vi "UnloadCrvEdPanel.vi"(8 "error in (no error)":errorcluster caption="entrée d'erreur (pas d'erreur)", 10 "CrvEdViRef":refnum<vi>, 11 "RemPanRef":refnum<vi>) -> (0 "error out":errorcluster caption="sortie d'erreur")   [LabVIEW 2019]
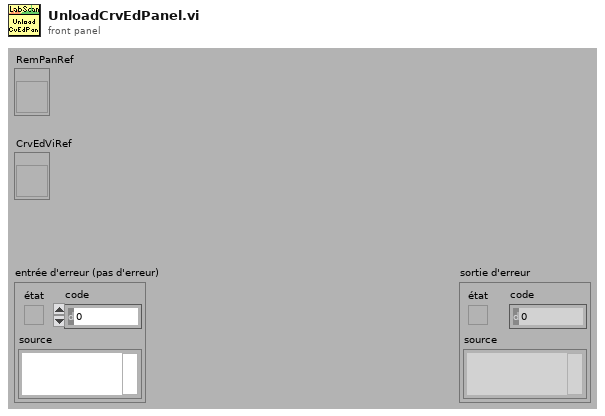
[diagram p1: front panel]
types:
  T1 = enum32{"Bad", "Idle", "Run top level", "Running"}
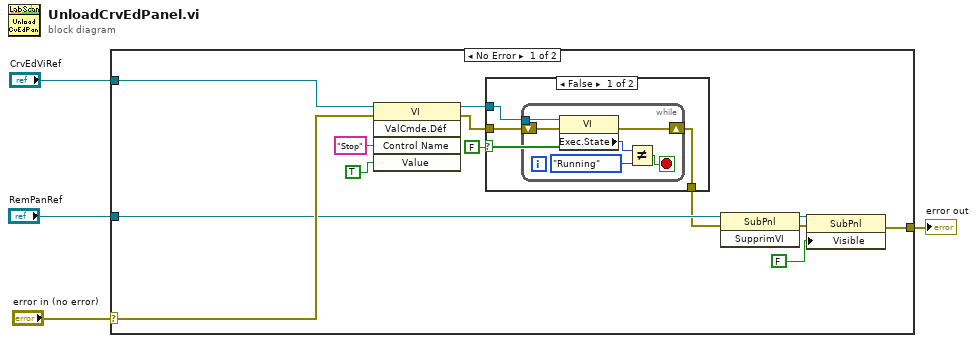
[diagram p0: block diagram]
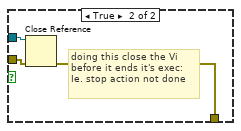
[diagram p2: hidden frame]
diagram:
  n1 = case shown="No Error" "error in (no error)" {
    selector: "error in (no error)" -> [w17 w30]
    tunnel: [w16 w30] -> w3
    tunnel: "RemPanRef" -> [w15 _]
    tunnel: "CrvEdViRef" -> [w14 _]
    frame No Error {
      n2 = invoke class="VI" method="ValCmde.Déf"(reference=w14, error in=w17, "Control Name"="Stop" ("Nom de la commande"), "Value"=TRUE) -> (reference out=w10:refnum<vi>, error out=w11:errorcluster)  [unwired: 1 in, 3 out]
      n3 = case shown="False" FALSE {
        tunnel: w11 -> [w19 w29]
        tunnel: w10 -> [w20 w28]
        tunnel: [w18 w27] -> w9
        frame False {
          n4 = while {
            tunnel: w20 -> [w26]
            shift-right: [w24] -> w18
            shift-left: w19 -> [w25]
            stop <- w21 stop-if-true
            n5 = property class="VI"(reference=w26, error in=w25) -> (error out=w24:errorcluster, "Exec.State"=w22:T1)  [unwired: 1 out]
            n6 = Not Equal?(x=w22, y=T1."Running" ("Exécution:État")) -> (x != y?=w21:bool)
          }
        }
        frame True {
          # "doing this close the Vi before it ends it's exec:\nIe. stop action not done"
          n7 = Close Reference(reference=w28, error in (no error)=w29) -> (error out=w27:errorcluster)
        }
      }
      n8 = invoke class="SubPnl" method="SupprimVI"(reference=w15, error in=w9) -> (reference out=w7:refnum<vi>, error out=w6:errorcluster)  [unwired: 1 in, 1 out]
      n9 = property class="SubPnl"(reference=w7, error in=w6, "Visible"=FALSE) -> (error out=w16:errorcluster)  [unwired: 1 out]
    }
    frame Error {
    }
  }
  "error out" <- w3
